vi "Adjust Reference Clock.vi"(0 "VISA resource name":refnum<visa-resource-name>, 5 "Adjust Reference Clock (511)":i32=511 min=0 max=1023, 7 "Reset Adjust Value (F:Disable)":bool, 11 "error in (no error)":errorcluster) -> (4 "VISA resource name out":refnum<visa-resource-name>, 15 "error out":errorcluster)   [LabVIEW 2020, in "Anritsu Signal Analyzer Series.lvlib"]
doc: "Sets the adjustment value for the internal reference signal oscillator (Reference Clock)."
uses:
  Anritsu Signal Analyzer Series.lvlib
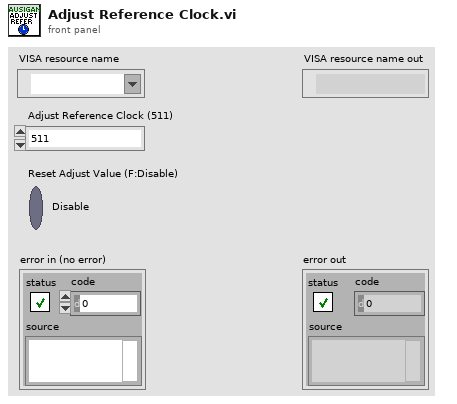
[diagram p1: front panel]
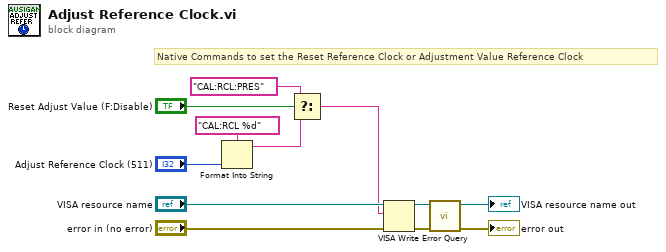
[diagram p0: block diagram]
diagram:
  # "Native Commands to set the Reset Reference Clock or Adjustment Value Reference Clock"
  n1 = Format Into String(format string="CAL:RCL %d" ("_CommandSet"), "Adjust Reference Clock (511)") -> (resulting string=w3:string)  [unwired: 2 in, 1 out]
  n2 = Select(t="CAL:RCL:PRES" ("_Command"), s="Reset Adjust Value (F:Disable)", f=w3) -> (s? t:f=w2:string)
  n3 = VISA Write(VISA resource name="VISA resource name", write buffer=w2, error in (no error)="error in (no error)") -> (VISA resource name out=w8:refnum<visa-resource-name>, error out=w7:errorcluster)  [unwired: 1 out]
  n4 = call "Error Query.vi"("error in (no error)"=w7, "VISA resource name"=w8) -> ("error out"=→"error out":errorcluster, "VISA resource name out"=→"VISA resource name out":refnum<visa-resource-name>)  [unwired: 6 in, 2 out]
